vi "testRmFileIfExist.vi"(8 "error in (no error)":errorcluster) -> (0 "error out":errorcluster)   [LabVIEW 2018]
uses:
  <vilib>/addons/_JKI Toolkits/Caraya/classes/Assert/Assert Not Error.vi
  <vilib>/addons/_JKI Toolkits/Caraya/classes/Assert/Assert False.vi
  <vilib>/addons/_JKI Toolkits/Caraya/classes/Test/Test.lvclass
  <vilib>/addons/_JKI Toolkits/Caraya/classes/Assert/Assert.lvclass
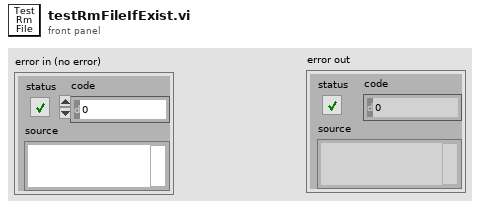
[diagram p1: front panel]
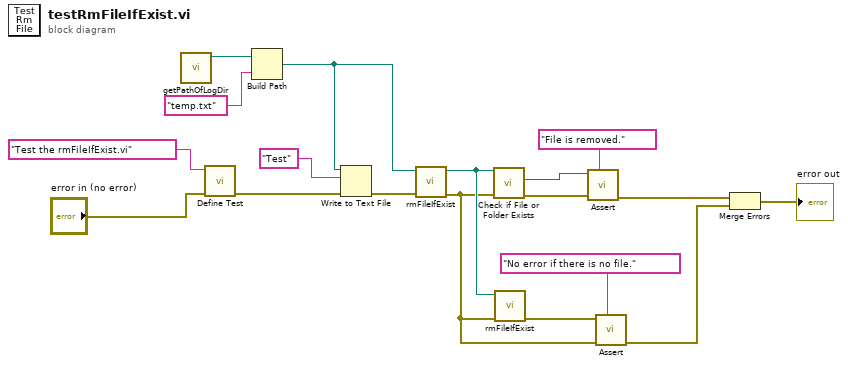
[diagram p0: block diagram]
diagram:
  n1 = call "getPathOfLogDir.vi"() -> ("logDirPath"=w16:path)  [unwired: 11 in]
  n2 = call <vilib>:"Define Test.vi"("error in (no error)"="error in (no error)", "Label (VI Title)"="Test the rmFileIfExist.vi") -> ("error out"=w14:errorcluster)  [unwired: 9 in]
  n3 = Build Path(base path=w16, name or relative path="temp.txt") -> (appended path=w11:path)
  n4 = Write to Text File(file (use dialog)=w11, text="Test", error in=w14) -> (error out=w12:errorcluster)  [unwired: 1 in, 2 out]
  n5 = call "rmFileIfExist.vi"("error in (no error)"=w12, "path"=w11) -> ("error out"=w5:errorcluster, "pathDup"=w7:path)  [unwired: 8 in]
  n6 = call <vilib>:"Check if File or Folder Exists.vi"("error in (no error)"=w5, "path"=w7) -> ("error out"=w10:errorcluster, "file or folder exists?"=w9:bool)  [unwired: 7 in, 1 out]
  n7 = call "rmFileIfExist.vi"("error in (no error)"=w5, "path"=w7) -> ("error out"=w6:errorcluster)  [unwired: 8 in, 1 out]
  n8 = call-poly <vilib>:"Assert.vi"("Label"="File is removed.", "error in (no error)"=w10, "False?"=w9) -> ("error out"=w3:errorcluster)  [unwired: 8 in]
  n9 = call-poly <vilib>:"Assert.vi"("Label"="No error if there is no file.", "error in (no error)"=w5, "Not Error?"=w6) -> ("error out"=w2:errorcluster)  [unwired: 8 in]
  n10 = Merge Errors(w3, w2) -> (→"error out":errorcluster)
